vi "Configure Arbitrary Waveform.vi"(4 "Frequency (1000 Hz)":dbl=1000.0, 6 "DC Offset (0 V)":dbl, 7 "Arbitrary Waveform Name (0: USER1)":u16(ring) items=["USER1", "USER2", "USER3", "USER4", "Edit Memory"], 8 "error in (no error)":errorcluster, 9 "Gain (1 V)":dbl=1.0, 10 "Channel (0: Channel 1)":u16(ring) items=["Channel 1", "Channel 2"], 11 "VISA resource name":refnum<visa-resource-name>) -> (0 "error out":errorcluster, 3 "VISA resource name out":refnum<visa-resource-name>)   [LabVIEW 2013, in "AWG.lvlib" / "Tektronix AFG 3000 Series.lvlib"]
doc: "Configures the function generator settings that affect arbitrary waveform generation."
uses:
  Tektronix AFG 3000 Series.lvlib
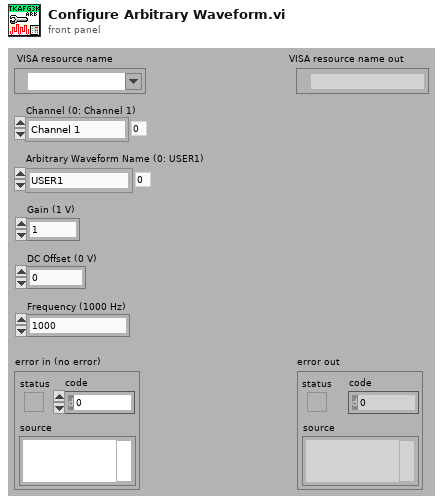
[diagram p1: front panel]
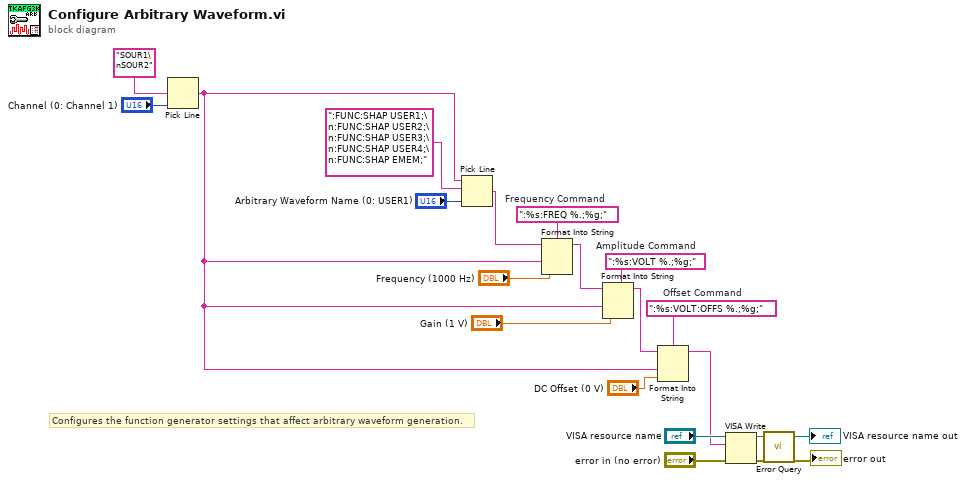
[diagram p0: block diagram]
diagram:
  w5 = ":%s:VOLT:OFFS %.;%g;"  # Offset Command
  w6 = ":%s:VOLT %.;%g;"  # Amplitude Command
  w7 = ":%s:FREQ %.;%g;"  # Frequency Command
  # "Configures the function generator settings that affect arbitrary waveform generation."
  n1 = Pick Line(multi-line string="SOUR1\nSOUR2" ("string (\"\")"), line index="Channel (0: Channel 1)") -> (output string=w1:string)  [unwired: 1 in]
  n2 = Pick Line(string ("")=w1, multi-line string=":FUNC:SHAP USER1;\n:FUNC:SHAP USER2;\n:FUNC:SHAP USER3;\n:FUNC:SHAP USER4;\n:FUNC:SHAP EMEM;" ("string (\"\")"), line index="Arbitrary Waveform Name (0: USER1)") -> (output string=w8:string)
  n3 = Format Into String(format string=w7, initial string=w8, w1, "Frequency (1000 Hz)") -> (resulting string=w12:string)  [unwired: 1 in, 1 out]
  n4 = Format Into String(format string=w6, initial string=w12, w1, "Gain (1 V)") -> (resulting string=w11:string)  [unwired: 1 in, 1 out]
  n5 = Format Into String(format string=w5, initial string=w11, w1, "DC Offset (0 V)") -> (resulting string=w15:string)  [unwired: 1 in, 1 out]
  n6 = VISA Write(VISA resource name="VISA resource name", write buffer=w15, error in (no error)="error in (no error)") -> (VISA resource name out=w19:refnum<visa-resource-name>, error out=w18:errorcluster)  [unwired: 1 out]
  n7 = call "Error Query.vi"("error in (no error)"=w18, "VISA resource name"=w19) -> ("error out"=→"error out":errorcluster, "VISA resource name out"=→"VISA resource name out":refnum<visa-resource-name>)  [unwired: 6 in, 2 out]
